vi "find all string constants.vi"   [LabVIEW 2012]
uses:
  <vilib>/Utility/traverseref.llb/TRef TravTarget.ctl
  <vilib>/Utility/traverseref.llb/VI Scripting - Traverse.lvlib
types:
  T1 = typedef "TRef TravTarget.ctl" = enum16{"FP", "BD", "Other"}
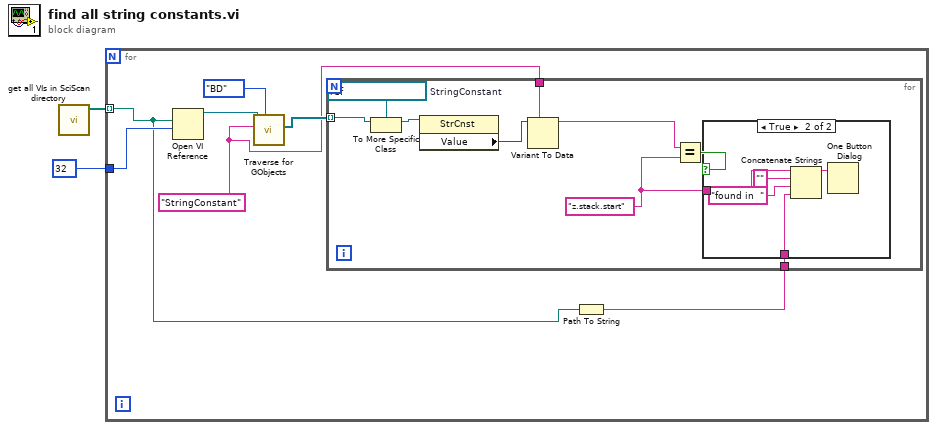
[diagram p0: block diagram]
diagram:
  n1 = call "get all VIs in SciScan directory.vi"() -> ("All Files in Dir"=w2:path[])  [unwired: 11 in]
  n2 = for {
    tunnel: w2 -> [w4] mode=indexing
    tunnel: 32 ("options") -> [w5]
    w6 = "StringConstant" ("Class Name")
    n3 = Open VI Reference(vi path=w4, options=w5) -> (vi reference=w9:refnum<vi>)  [unwired: 4 in, 1 out]
    n4 = call <vilib>:"Traverse for GObjects.vi"("Traverse Target"=TRef_TravTarget."BD", "Class Name"=w6, "VI Refnum"=w9) -> ("References"=w7:refnum<vi>[])  [unwired: 5 in, 3 out]
    n5 = Path To String(path=w4) -> (string=w3:string)
    n6 = for {
      tunnel: w7 -> [w18] mode=indexing
      tunnel: w6 -> [w14]
      tunnel: w3 -> [w10]
      w11 = "z.stack.start"
      w17 = refnum<vi> refnum  # StringConstant
      n7 = To More Specific Class(target class=w17, reference=w18) -> (specific class reference=w16:refnum<vi>)  [unwired: 1 in, 1 out]
      n8 = property class="StrCnst"(reference=w16) -> ("Value"=w15:variant)  [unwired: 1 in, 2 out]
      n9 = Variant To Data(type=w14, Variant=w15) -> (data=w13:string)  [unwired: 1 in, 1 out]
      n10 = Equal?(x=w13, y=w11) -> (x = y?=w12:bool)
      n11 = case shown="True" w12 {
        tunnel: w11 -> [_ w22]
        tunnel: w10 -> [_ w19]
        frame False {
        }
        frame True {
          n12 = Concatenate Strings(w22, "" ("string"), "found in  " ("string"), w19) -> (w23:string)
          n13 = One Button Dialog(message=w23) -> ()  [unwired: 1 in, 1 out]
        }
      }
    }
  }
